vi "PMX_AssignLimitSwitch.vi"(8 "Error in":errorcluster, 10 "LimitSwitch":T1, 11 "Device":refnum<k24>) -> (0 "Error out":errorcluster, 2 "Result":bool, 3 "Device":refnum<k24>)   [LabVIEW 2016]
doc: "Assigns LimitSwitch settings to the given device \nIf a limit switch with an already in use LimitSwitchNumber is assigned, that existing limit switch will be overwritten.\n\nResult: True, if assignment was successful, otherwise false\n\nLimitSwitchNumber: Number of the limit to assign (1..32)\nLimitSwitch:\nEnabled: Determines if limit switch operation is activated. \nHysteresis:Hysteresis value. Dependents on OperationDirection, it may also be used to define the band span. \nIgnoreMeasurementValueStatus: Determines if the status of the measurement value is ignored during evaluation of limit switch status.\nInputSignal: Signal whose measurement value is used to evaluate the limit switch. \nInvertResetBehaviour: If true, the defined ResetBehavior is inverted. \nLimit: Limit value. Dependents on OperationDirection, it may also be used to define the lower band value. \nLimitSwitchNumber: Number of the limit switch. This can range from 1 to 32. \nOperatingDirection: Operation direction of the limit switch. \nResetBehaviorMask: Reset behavior. Binary mask which is ANDed with all digital inputs. The reset behavior can be inverted with InvertResetBehavior. Default setting is 0."
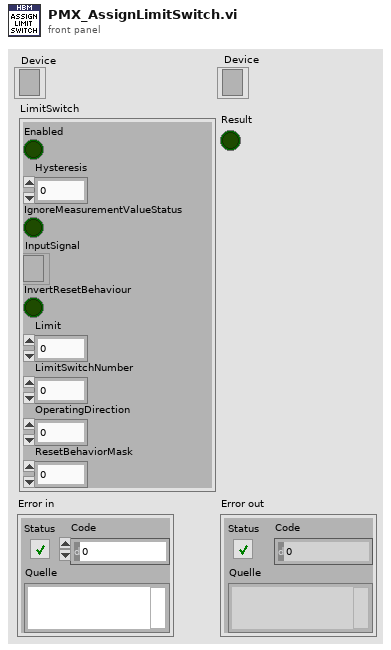
[diagram p1: front panel]
types:
  T1 = cluster{"Enabled":bool, "Hysteresis":dbl, "IgnoreMeasurementValueStatus":bool, "InputSignal":refnum<k24>, "InvertResetBehaviour":bool, "Limit":dbl, "LimitSwitchNumber":i32, "OperatingDirection":i32, "ResetBehaviorMask":i32}
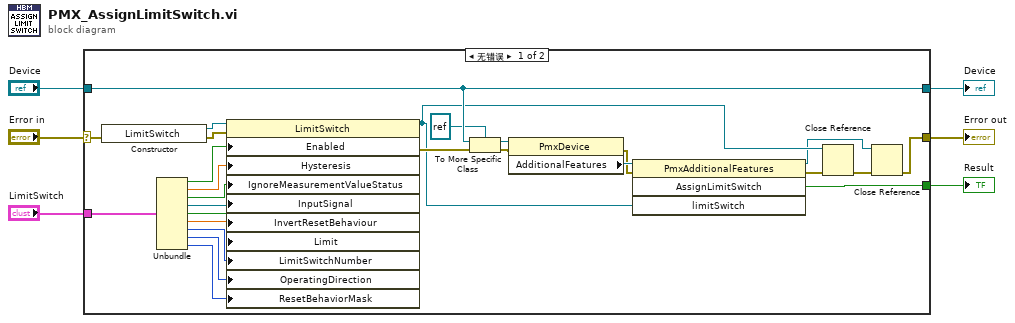
[diagram p0: block diagram]
diagram:
  n1 = case shown="无错误" "Error in" {
    selector: "Error in" -> [w15 w34]
    tunnel: [w7 w34] -> w4
    tunnel: "Device" -> [w17 w33]
    tunnel: [w17 w33] -> w5
    tunnel: "LimitSwitch" -> [w27 _]
    tunnel: [w16 _] -> w1
    frame No Error {
      n2 = constructor class="LimitSwitch"(error in=w15) -> (reference out=w28:refnum<k24>, error out=w14:errorcluster)  [unwired: 2 in, 1 out]
      n3 = Unbundle(w27) -> ("Enabled"=w26:bool, "Hysteresis"=w25:dbl, "IgnoreMeasurementValueStatus"=w24:bool, "InputSignal"=w23:refnum<k24>, "InvertResetBehaviour"=w22:bool, "Limit"=w21:dbl, "LimitSwitchNumber"=w20:i32, "OperatingDirection"=w19:i32, "ResetBehaviorMask"=w18:i32)
      n4 = property on="Eigenschaftsknoten" class="LimitSwitch"(reference=w28, error in=w14, "Enabled"=w26, "Hysteresis"=w25, "IgnoreMeasurementValueStatus"=w24, "InputSignal"=w23, "InvertResetBehaviour"=w22, "Limit"=w21, "LimitSwitchNumber"=w20, "OperatingDirection"=w19, "ResetBehaviorMask"=w18) -> (reference out=w9:refnum<k24>, error out=w13:errorcluster)
      n5 = To More Specific Class(target class=refnum<k24> refnum ("Zielklasse"), reference=w17, error in=w13) -> (specific class reference=w32:refnum<k24>, error out=w29:errorcluster)
      n6 = property on="Eigenschaftsknoten" class="PmxDevice"(reference=w32, error in=w29) -> (error out=w30:errorcluster, "AdditionalFeatures"=w31:refnum<k24>)  [unwired: 1 out]
      n7 = invoke on="Methodenknoten" class="PmxAdditionalFeatures" method="AssignLimitSwitch"(reference=w31, error in=w30, "limitSwitch"=w9) -> (reference out=w8:refnum<k24>, error out=w11:errorcluster, "AssignLimitSwitch"=w16:bool)  [unwired: 1 in, 1 out]
      n8 = Close Reference(reference=w9, error in (no error)=w11) -> (error out=w10:errorcluster)
      n9 = Close Reference(reference=w8, error in (no error)=w10) -> (error out=w7:errorcluster)
    }
    frame Error {
    }
  }
  "Device" <- w5
  "Error out" <- w4
  "Result" <- w1
